vi "Test Server.vi"   [LabVIEW 2013]
uses:
  Message Queue/ctl_MessageQueue.ctl
  Message Queue/Message Queue.lvlib
  WebSockets/WebSockets.lvlib
types:
  T1 = typedef "Message Queue.lvlib/ctl_MessageQueue.ctl" = cluster{"Command":string, "Data":variant}
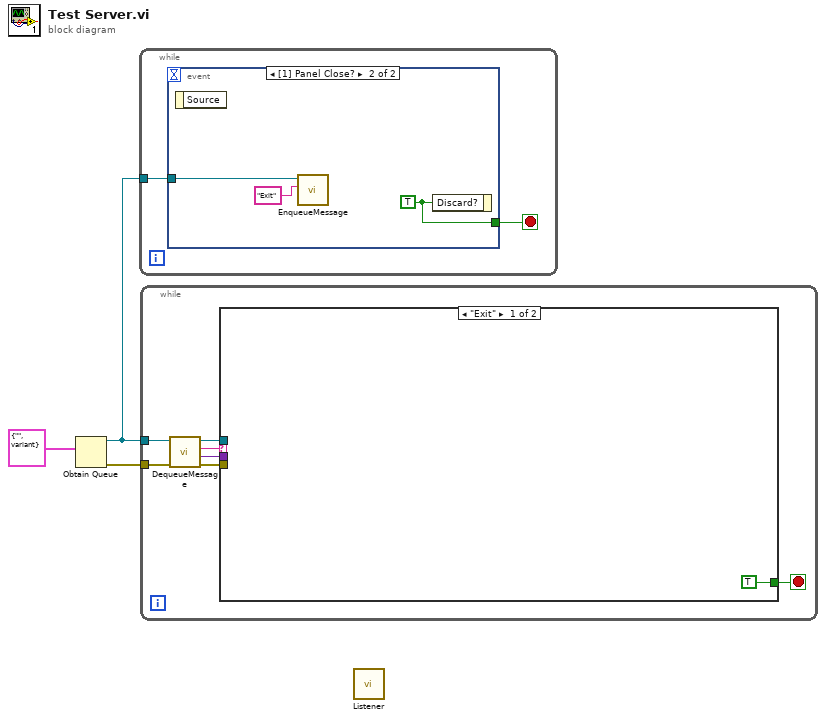
[diagram p0: block diagram]
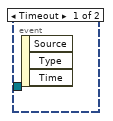
[diagram p3: hidden frame]
diagram:
  n1 = Obtain Queue(element data type=T1 {"Command"="", "Data"=variant}) -> (queue out=w1:refnum<queue>, error out=w2:errorcluster)  [unwired: 4 in, 1 out]
  n2 = while {
    tunnel: w1 -> [w5]
    stop <- w4 stop-if-true
    n3 = event shown="[1] Panel Close?" {
      selector: _ -> [_ _]
      dyn-events: _ -> [_ _]
      timeout: _ -> [_ _]
      tunnel: w5 -> [_ w8]
      tunnel: [_ w6] -> w4
      event Timeout {
        n4 = event-data() -> ()  [unwired: 1 in, 3 out]
      }
      event Panel Close? {
        w6 = TRUE ("Discard?")
        n5 = event-data() -> ()  [unwired: 1 in, 1 out]
        n6 = call "EnqueueMessage.vi"("Command"="Exit", "Queue in"=w8) -> ()  [unwired: 8 in, 2 out]
        n7 = event-data("Discard?"=w6) -> ()  [unwired: 1 in, 1 out]
      }
    }
  }
  n8 = while {
    tunnel: w2 -> [w11]
    tunnel: w1 -> [w10]
    stop <- w15 stop-if-true
    n9 = call "DequeueMessage.vi"("error in (no error)"=w11, "Message Queue In"=w10) -> ("error out"=w12:errorcluster, "Data"=w13:variant, "Command"=w14:string, "Message Queue Out"=w9:refnum<queue>)  [unwired: 6 in]
    n10 = case shown="\"Exit\"" w14 {
      tunnel: [TRUE _] -> w15
      tunnel: w13 -> [_ _]
      tunnel: w12 -> [_ _]
      tunnel: w9 -> [_ _]
      frame "Exit" {
      }
      frame Default {
      }
    }
  }
  n11 = call "Listener.vi"() -> ()  [unwired: 12 in]
